vi "WAPIAerScopeDump.vi"(3 "count":u16, 9 "error in (no error)":errorcluster) -> (0 "scopebuf":i32[](array[numeric]), 2 "firstdata":i32, 6 "error out":errorcluster)   [LabVIEW 2009]
uses:
  win50032.dll
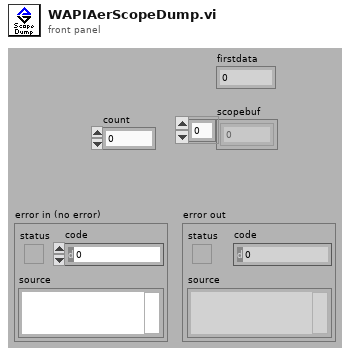
[diagram p1: front panel]
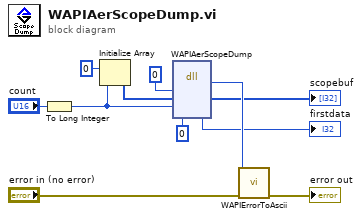
[diagram p0: block diagram]
diagram:
  n1 = To Long Integer(number="count") -> (32bit integer=w1:i32)
  n2 = Initialize Array(0 ("timeout"), w1) -> (w3:i32[])
  n3 = dll-call lib="Win50032.dll" fn="WAPIAerScopeDump"("timeout"=0, "scopebuf"=w3, "count"=w1, "firstdata"=0) -> ("return type"=w9:u32, "scopebuf"=→"scopebuf":i32[], "firstdata"=→"firstdata":i32)  [unwired: 5 in, 2 out]
  n4 = call "WAPIErrorToAscii.vi"("error in (no error)"="error in (no error)", "error"=w9) -> ("error out"=→"error out":errorcluster)  [unwired: 8 in, 1 out]
